vi "LEDs_manager.vi"(8 "Error In":errorcluster) -> (0 "Error Out":errorcluster)   [LabVIEW 2013]
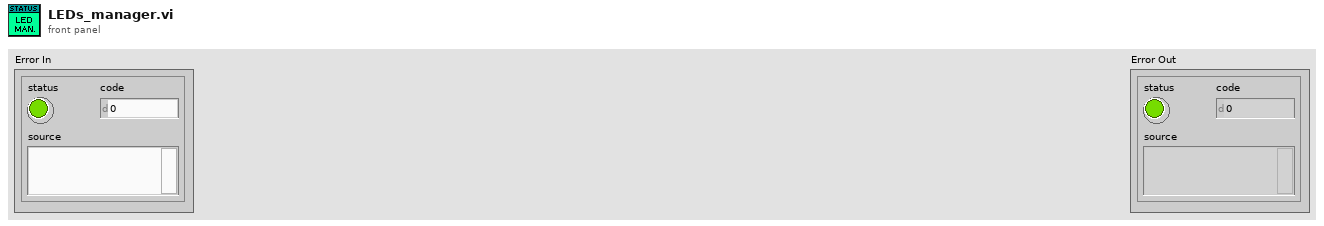
[diagram p1: front panel]
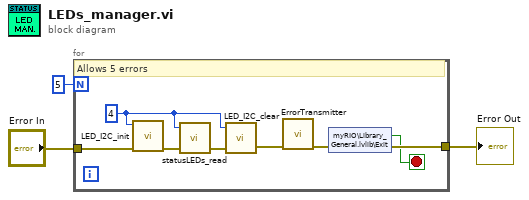
[diagram p0: block diagram]
diagram:
  n1 = for {
    N: 5 -> [_]
    tunnel: "Error In" -> [w8]
    tunnel: [w5] -> w2
    stop <- w4 stop-if-true
    w11 = u8 4 ("SCI")
    # "Allows 5 errors"
    n2 = call "LED_I2C_init.vi"("Error In"=w8, "Servo Controller Index"=w11) -> ("Error Out"=w10:errorcluster)  [unwired: 9 in]
    n3 = call "statusLEDs_read.vi"("error in (no error)"=w10, "SCI"=w11) -> ("Error Out"=w9:errorcluster)  [unwired: 3 in]
    n4 = call "LED_I2C_clear.vi"("Error In"=w9, "Servo Controller Index"=w11) -> ("Error Out"=w7:errorcluster)  [unwired: 2 in]
    n5 = call "ErrorTransmitter.vi"("Error In"=w7) -> ("Error Out"=w6:errorcluster)  [unwired: 10 in]
    n6 = shared-variable "myRIO\\Library_General.lvlib\\Exit"(error in=w6) -> (w4:bool, error out=w5:errorcluster)
  }
  "Error Out" <- w2
